vi "check_PE.vi"(3 "error in (no error)":errorcluster, 4 "\\lambda":dbl, 5 "phi(t)":T1, 6 "\\Sigma (phi) (phi)^T (t-1)":T1) -> (0 "error out":errorcluster, 1 "x > y?":bool, 2 "\\Sigma (\\phi) (\\phi)^T (t)":T1)   [LabVIEW 2021]
uses:
  <vilib>/Analysis/Matrix/Datatypes/RealMatrix.ctl
  <vilib>/Analysis/7linalg.llb/Eigenvalue and Vectors Output Option.ctl
  <vilib>/Analysis/Matrix/Numeric/Multiply/Multiply - RM,RM.vi
  <vilib>/Analysis/Matrix/Numeric/Multiply/Multiply - R,RM.vi
  <vilib>/Analysis/Matrix/Numeric/Add/Add - RM,RM.vi
  <vilib>/Analysis/7linalg.llb/Real Eigenvalues and Vectors.vi
  <vilib>/Analysis/Matrix/NI_Matrix.lvlib
  <vilib>/Analysis/NI_AALPro.lvlib
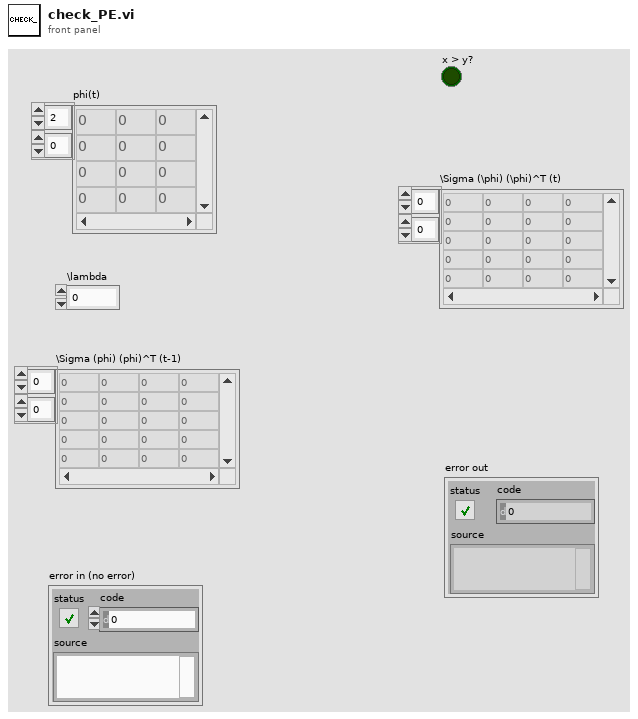
[diagram p1: front panel]
types:
  T1 = typedef "NI_Matrix.lvlib/RealMatrix.ctl" = dbl[][]
  T2 = typedef "NI_AALPro.lvlib/Eigenvalue and Vectors Output Option.ctl" = i32
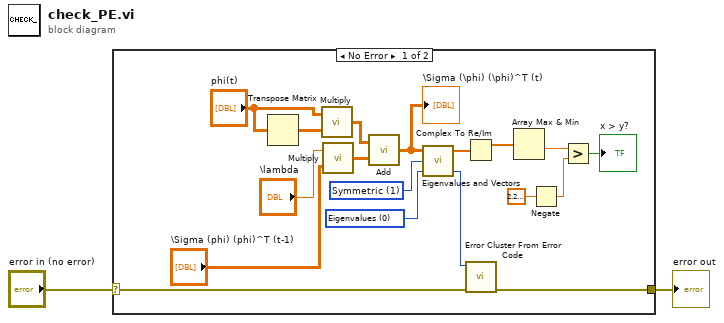
[diagram p0: block diagram]
diagram:
  n1 = case shown="No Error" "error in (no error)" {
    selector: "error in (no error)" -> [w4 w21]
    tunnel: [w3 w21] -> w1
    frame No Error {
      w14 = 1 items=["General", "Symmetric"] ("matrix type")
      w15 = T2 0 items=["Eigenvalues", "Eigenvalues & Vectors"] ("output option")
      n2 = Transpose Matrix(1:"phi(t)") -> (0:w19:T1)
      n3 = call-poly <vilib>:"Multiply.vi"("Real Matrix B"=w19, "Real Matrix A"="phi(t)") -> ("A * B"=w18:T1)
      n4 = call-poly <vilib>:"Multiply.vi"("Real Matrix A"="\\Sigma (phi) (phi)^T (t-1)", "Real Scalar c"="\\lambda") -> ("c * A"=w16:T1)
      n5 = call-poly <vilib>:"Add.vi"("Real Matrix B"=w16, "Real Matrix A"=w18) -> ("A + B"=w11:T1)
      "\\Sigma (\\phi) (\\phi)^T (t)" <- w11
      n6 = call-poly <vilib>:"Eigenvalues and Vectors.vi"("output option"=w15, "matrix type"=w14, "Input Matrix"=w11) -> ("error"=w5:i32, "Eigenvalues"=w13:cdb[])  [unwired: 1 out]
      n7 = Complex To Re/Im(x + iy=w13) -> (x=w10:dbl[])  [unwired: 1 out]
      n8 = call <vilib>:"Error Cluster From Error Code.vi"("error in (no error)"=w4, "error code (0)"=w5) -> ("error out"=w3:errorcluster)  [unwired: 7 in]
      n9 = Array Max & Min(array=w10) -> (min value=w9:dbl)  [unwired: 3 out]
      n10 = Negate(x=2.220446049250313e-16) -> (-x=w7:dbl)
      n11 = Greater?(x=w9, y=w7) -> (0:→"x > y?":bool)
    }
    frame Error {
    }
  }
  "error out" <- w1
